vi "Apply Tournaments Played Threshold.vi"(10 "Tournaments Played  Threshold":u32, 11 "Raw WPC Player Stats":T1(array[cluster])) -> (3 "Filtered Stats":T1(array[cluster]))   [LabVIEW 2020]
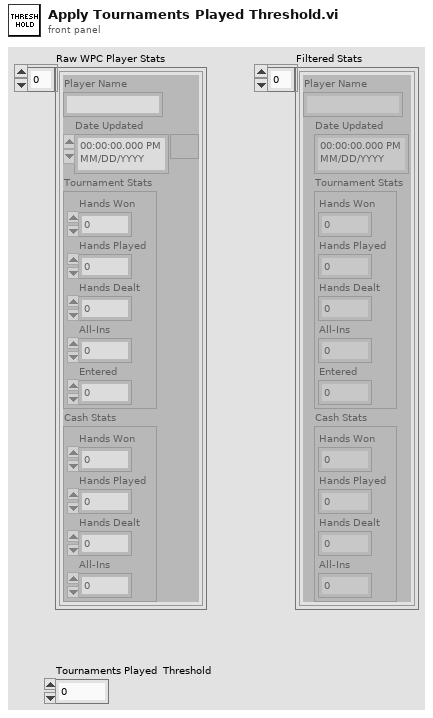
[diagram p1: front panel]
types:
  T1 = cluster{"Player Name":string, "Date Updated":timestamp, "Tournament Stats":cluster{"Hands Won":dbl, "Hands Played":dbl, "Hands Dealt":dbl, "All-Ins":dbl, "Entered":dbl}, "Cash Stats":cluster{"Hands Won":dbl, "Hands Played":dbl, "Hands Dealt":dbl, "All-Ins":dbl}}[]
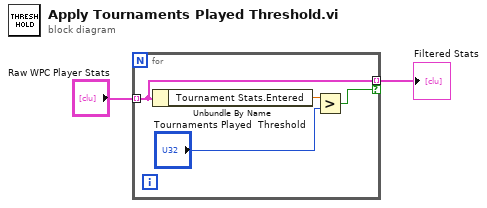
[diagram p0: block diagram]
diagram:
  n1 = for {
    tunnel: "Raw WPC Player Stats" -> [w4] mode=indexing
    tunnel: [w4] -> w2 mode=indexing if=w3
    n2 = Unbundle By Name(w4) -> ("Tournament Stats.Entered"=w6:dbl)
    n3 = Greater?(x=w6, y="Tournaments Played  Threshold") -> (0:w3:bool)
  }
  "Filtered Stats" <- w2
